vi "testGetCscIndex.vi"(8 "error in (no error)":errorcluster) -> (0 "error out":errorcluster)   [LabVIEW 2018]
uses:
  src/SalProcess/SalProcess.lvclass
  <vilib>/addons/_JKI Toolkits/Caraya/classes/Assert/Assert Equal Value_Variant.vi
  <vilib>/addons/_JKI Toolkits/Caraya/classes/Test/Test.lvclass
  <vilib>/addons/_JKI Toolkits/Caraya/classes/Assert/Assert.lvclass
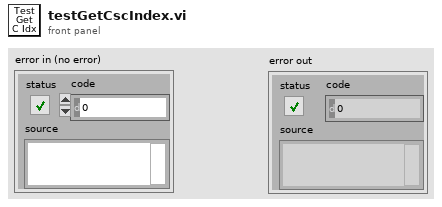
[diagram p1: front panel]
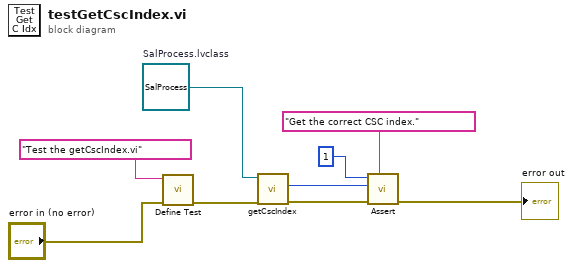
[diagram p0: block diagram]
diagram:
  w7 = refnum<class "SalProcess.lvclass"> refnum  # SalProcess.lvclass
  n1 = call <vilib>:"Define Test.vi"("error in (no error)"="error in (no error)", "Label (VI Title)"="Test the getCscIndex.vi") -> ("error out"=w6:errorcluster)  [unwired: 9 in]
  n2 = call "getCscIndex.vi"("error in (no error)"=w6, "SalProcess in"=w7) -> ("error out"=w5:errorcluster, "cscIdx"=w4:i32)  [unwired: 7 in, 1 out]
  n3 = call-poly <vilib>:"Assert.vi"("Label"="Get the correct CSC index." ("Label (VI Title)"), "error in (no error)"=w5, "Y"=w4, "X"=1 ("cscIdx")) -> ("error out"=→"error out":errorcluster)  [unwired: 7 in]
